vi "Andor_iXon_Init.vi"(8 "error in (no error)":errorcluster, 11 "input cluster":T6) -> (0 "error out":errorcluster)   [LabVIEW 2009]
uses:
  atmcd32d.llb/AcquisitionMode_mode typedef.ctl
  atmcd32d.llb/FanMode_mode typedef.ctl
  atmcd32d.llb/ReadMode_mode typedef.ctl
  atmcd32d.llb/TriggerMode_mode typedef.ctl
  atmcd32d.llb/Shutter_type typedef.ctl
  atmcd32d.llb/Shutter_mode typedef.ctl
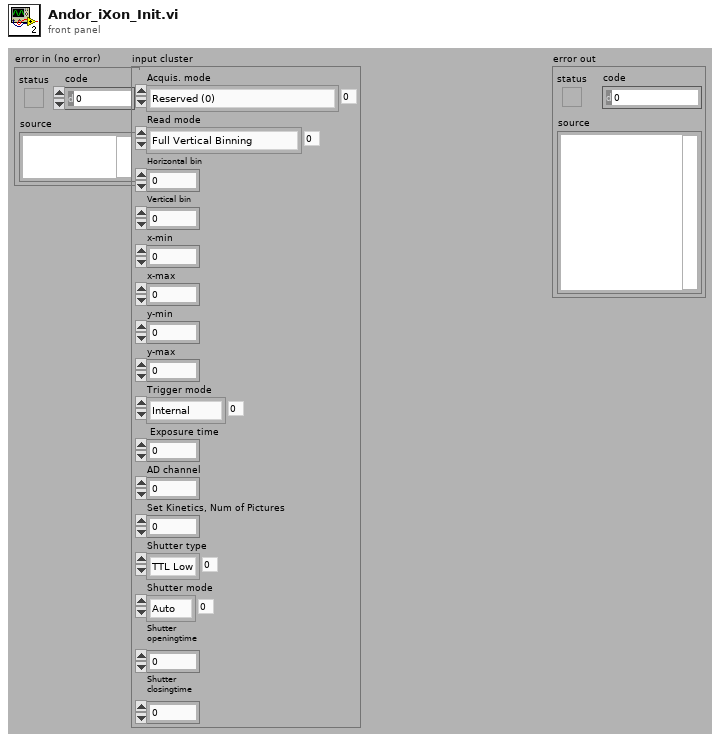
[diagram p1: front panel]
types:
  T1 = typedef "AcquisitionMode_mode typedef.ctl" = enum16{"Reserved (0)", "Single Scan", "Accumulate", "Kinetics", "Fast Kinetics", "Run Till Abort", "Reserved (6)", "Reserved (7)", "Reserved (8)", "Time Delayed Integration"}
  T2 = typedef "ReadMode_mode typedef.ctl" = enum16{"Full Vertical Binning", "Multi-Track", "Random-Track", "Single-Track", "Image"}
  T3 = typedef "TriggerMode_mode typedef.ctl" = enum16{"Internal", "External", "N/A (2)", "N/A (3)", "N/A (4)", "N/A (5)", "External Start"}
  T4 = typedef "Shutter_type typedef.ctl" = enum16{"TTL Low", "TTL High"}
  T5 = typedef "Shutter_mode typedef.ctl" = enum16{"Auto", "Open", "Close"}
  T6 = cluster{"Acquis. mode":T1, "Read mode":T2, "Horizontal bin":i32, "Vertical bin":i32, "x-min":i32, "x-max":i32, "y-min":i32, "y-max":i32, "Trigger mode":T3, " Exposure time":sgl, "AD channel":i32, "Set Kinetics, Num of Pictures":i32, "Shutter type":T4, "Shutter mode":T5, "Shutter\nopeningtime":i32, "Shutter\nclosingtime":i32}
  T7 = typedef "FanMode_mode typedef.ctl" = enum16{"fan on full", "fan on low", "fan off"}
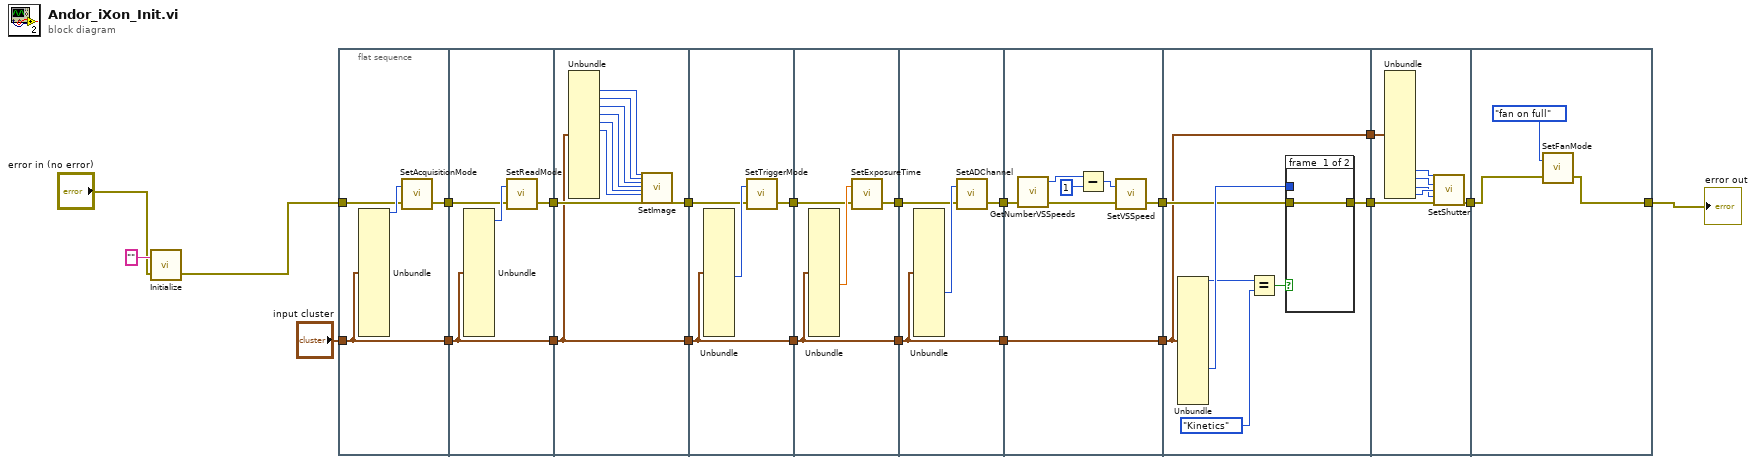
[diagram p0: block diagram]
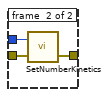
[diagram p2: hidden frame]
diagram:
  n1 = call "Initialize.vi"("error in (no error)"="error in (no error)", "directory (\"\")"="") -> ("error out"=w2:errorcluster)  [unwired: 1 out]
  n2 = flat-sequence {
    tunnel: "input cluster" -> [w25]
    tunnel: [w25] -> w20
    tunnel: w2 -> [w24]
    tunnel: [w23] -> w19
    tunnel: w20 -> [w27]
    tunnel: [w27] -> w18
    tunnel: w19 -> [w29]
    tunnel: [w28] -> w17
    tunnel: w18 -> [w35]
    tunnel: [w35] -> w16
    tunnel: w17 -> [w39]
    tunnel: [w38] -> w15
    tunnel: w16 -> [w40]
    tunnel: [w40] -> w14
    tunnel: w15 -> [w42]
    tunnel: [w41] -> w13
    tunnel: w14 -> [w44]
    tunnel: [w44] -> w12
    tunnel: w13 -> [w46]
    tunnel: [w45] -> w11
    tunnel: w12 -> [w48]
    tunnel: [w48] -> w10
    tunnel: w11 -> [w50]
    tunnel: [w49] -> w9
    tunnel: w10 -> [w52]
    tunnel: [w52] -> w8
    tunnel: w9 -> [w55]
    tunnel: [w53] -> w7
    tunnel: w8 -> [w62]
    tunnel: [w62] -> w6
    tunnel: w7 -> [w64]
    tunnel: [w63] -> w5
    tunnel: w6 -> [w70]
    tunnel: w5 -> [w72]
    tunnel: [w71] -> w1
    tunnel: [w77] -> w22
    tunnel: w1 -> [w78]
    frame #0 {
      n3 = Unbundle(w25) -> ("Acquis. mode"=w26:T1)  [unwired: 15 out]
      n4 = call "SetAcquisitionMode.vi"("error in (no error)"=w24, "mode"=w26) -> ("error out"=w23:errorcluster)  [unwired: 1 out]
    }
    frame #1 {
      n5 = Unbundle(w27) -> ("Read mode"=w30:T2)  [unwired: 15 out]
      n6 = call "SetReadMode.vi"("error in (no error)"=w29, "mode"=w30) -> ("error out"=w28:errorcluster)  [unwired: 1 out]
    }
    frame #2 {
      n7 = Unbundle(w35) -> ("Horizontal bin"=w37:i32, "Vertical bin"=w36:i32, "x-min"=w34:i32, "x-max"=w33:i32, "y-min"=w32:i32, "y-max"=w31:i32)  [unwired: 10 out]
      n8 = call "SetImage.vi"("hbin"=w37, "vbin"=w36, "hstart"=w34, "hend"=w33, "vstart"=w32, "vend"=w31, "error in (no error)"=w39) -> ("error out"=w38:errorcluster)  [unwired: 20 out]
    }
    frame #3 {
      n9 = Unbundle(w40) -> ("Trigger mode"=w43:T3)  [unwired: 15 out]
      n10 = call "SetTriggerMode.vi"("error in (no error)"=w42, "mode"=w43) -> ("error out"=w41:errorcluster)  [unwired: 1 out]
    }
    frame #4 {
      n11 = Unbundle(w44) -> ("Exposure time"=w47:sgl)  [unwired: 15 out]
      n12 = call "SetExposureTime.vi"("error in (no error)"=w46, "time"=w47) -> ("error out"=w45:errorcluster)  [unwired: 1 out]
    }
    frame #5 {
      n13 = Unbundle(w48) -> ("AD channel"=w51:i32)  [unwired: 15 out]
      n14 = call "SetADChannel.vi"("error in (no error)"=w50, "channel"=w51) -> ("error out"=w49:errorcluster)  [unwired: 1 out]
    }
    frame #6 {
      n15 = call "GetNumberVSSpeeds.vi"("error in (no error)"=w55) -> ("error out"=w54:errorcluster, "number"=w56:i32)  [unwired: 3 out]
      n16 = Subtract(x=w56, y=1) -> (x-y=w58:i32)
      n17 = call "SetVSSpeed.vi"("error in (no error)"=w54, "index"=w58) -> ("error out"=w53:errorcluster)  [unwired: 1 out]
    }
    frame #7 {
      n18 = Unbundle(w62) -> ("Acquis. mode"=w61:T1, "Set Kinetics, Num of Pictures"=w65:i32)  [unwired: 14 out]
      n19 = Equal?(x=w61, y=AcquisitionMode_mode_typedef."Kinetics") -> (x = y?=w59:bool)
      n20 = case shown="False" w59 {
        tunnel: w65 -> [_ w69]
        tunnel: w64 -> [w66 w68]
        tunnel: [w66 w67] -> w63
        frame #0 {
        }
        frame #1 {
          n21 = call "SetNumberKinetics.vi"("error in (no error)"=w68, "number"=w69) -> ("error out"=w67:errorcluster)  [unwired: 1 out]
        }
      }
    }
    frame #8 {
      n22 = Unbundle(w70) -> ("Shutter type"=w73:T4, "Shutter mode"=w74:T5, "Shutter\nopeningtime"=w75:i32, "Shutter\nclosingtime"=w76:i32)  [unwired: 12 out]
      n23 = call "SetShutter.vi"("type"=w73, "mode"=w74, "closingtime"=w76, "openingtime"=w75, "error in (no error)"=w72) -> ("error out"=w71:errorcluster)  [unwired: 10 out]
    }
    frame #9 {
      n24 = call "SetFanMode.vi"("error in (no error)"=w78, "mode"=FanMode_mode_typedef."fan on full") -> ("error out"=w77:errorcluster)  [unwired: 1 out]
    }
  }
  "error out" <- w22
